vi "CT traits extraction_Maize stem_English version.vi"() -> ()   [LabVIEW 2015]
uses:
  <vilib>/Utility/file.llb/Write Delimited Spreadsheet (DBL).vi
  <vilib>/vision/NI_Vision_Development_Module.lvlib
  <vilib>/Utility/file.llb/Read From Spreadsheet File (string).vi
  CTThickness.dll
panel:
  out "Numeric":i32
  in  "Path of data storage":path=path "E:/文章投稿/51. 代明球老师-玉米胁迫实验/CT程序/section-test/results.txt"
  out "appended path":path
  in  "Path of reconstructed images":path=path "E:/文章投稿/51. 代明球老师-玉米胁迫实验/CT程序/section-test"
  out "Duty_cycle":dbl
  out "Cavity_area":dbl
  out "Hollow_area":dbl
  out "Vascular_area":dbl
  out "8. 维管束小区域图":T1(plugin-control)
  out "7. 维管束闭操作":T1(plugin-control)
  out "6. Vascular image":T1(plugin-control)
  out "5. Hollow grayscale image":T1(plugin-control)
  out "Culm_area":sgl
  out "Culm_wall_area":sgl
  out "Major_axis":sgl
  out "Minor_axis":sgl
  out "4. Hollow binary image":T1(plugin-control)
  out "Culm_diameter":sgl
  out "3. Culm wall image":T1(plugin-control)
  in  "图片路径 2":path=path "E:/文章投稿/51. 代明球老师-玉米胁迫实验/CT程序/CTThickness_2/空图.png"
  out "2. Culm wall image":T1(plugin-control)
  out "Wall_thickness":sgl
  out "1. Reconstructed transverse section images":T1(plugin-control)
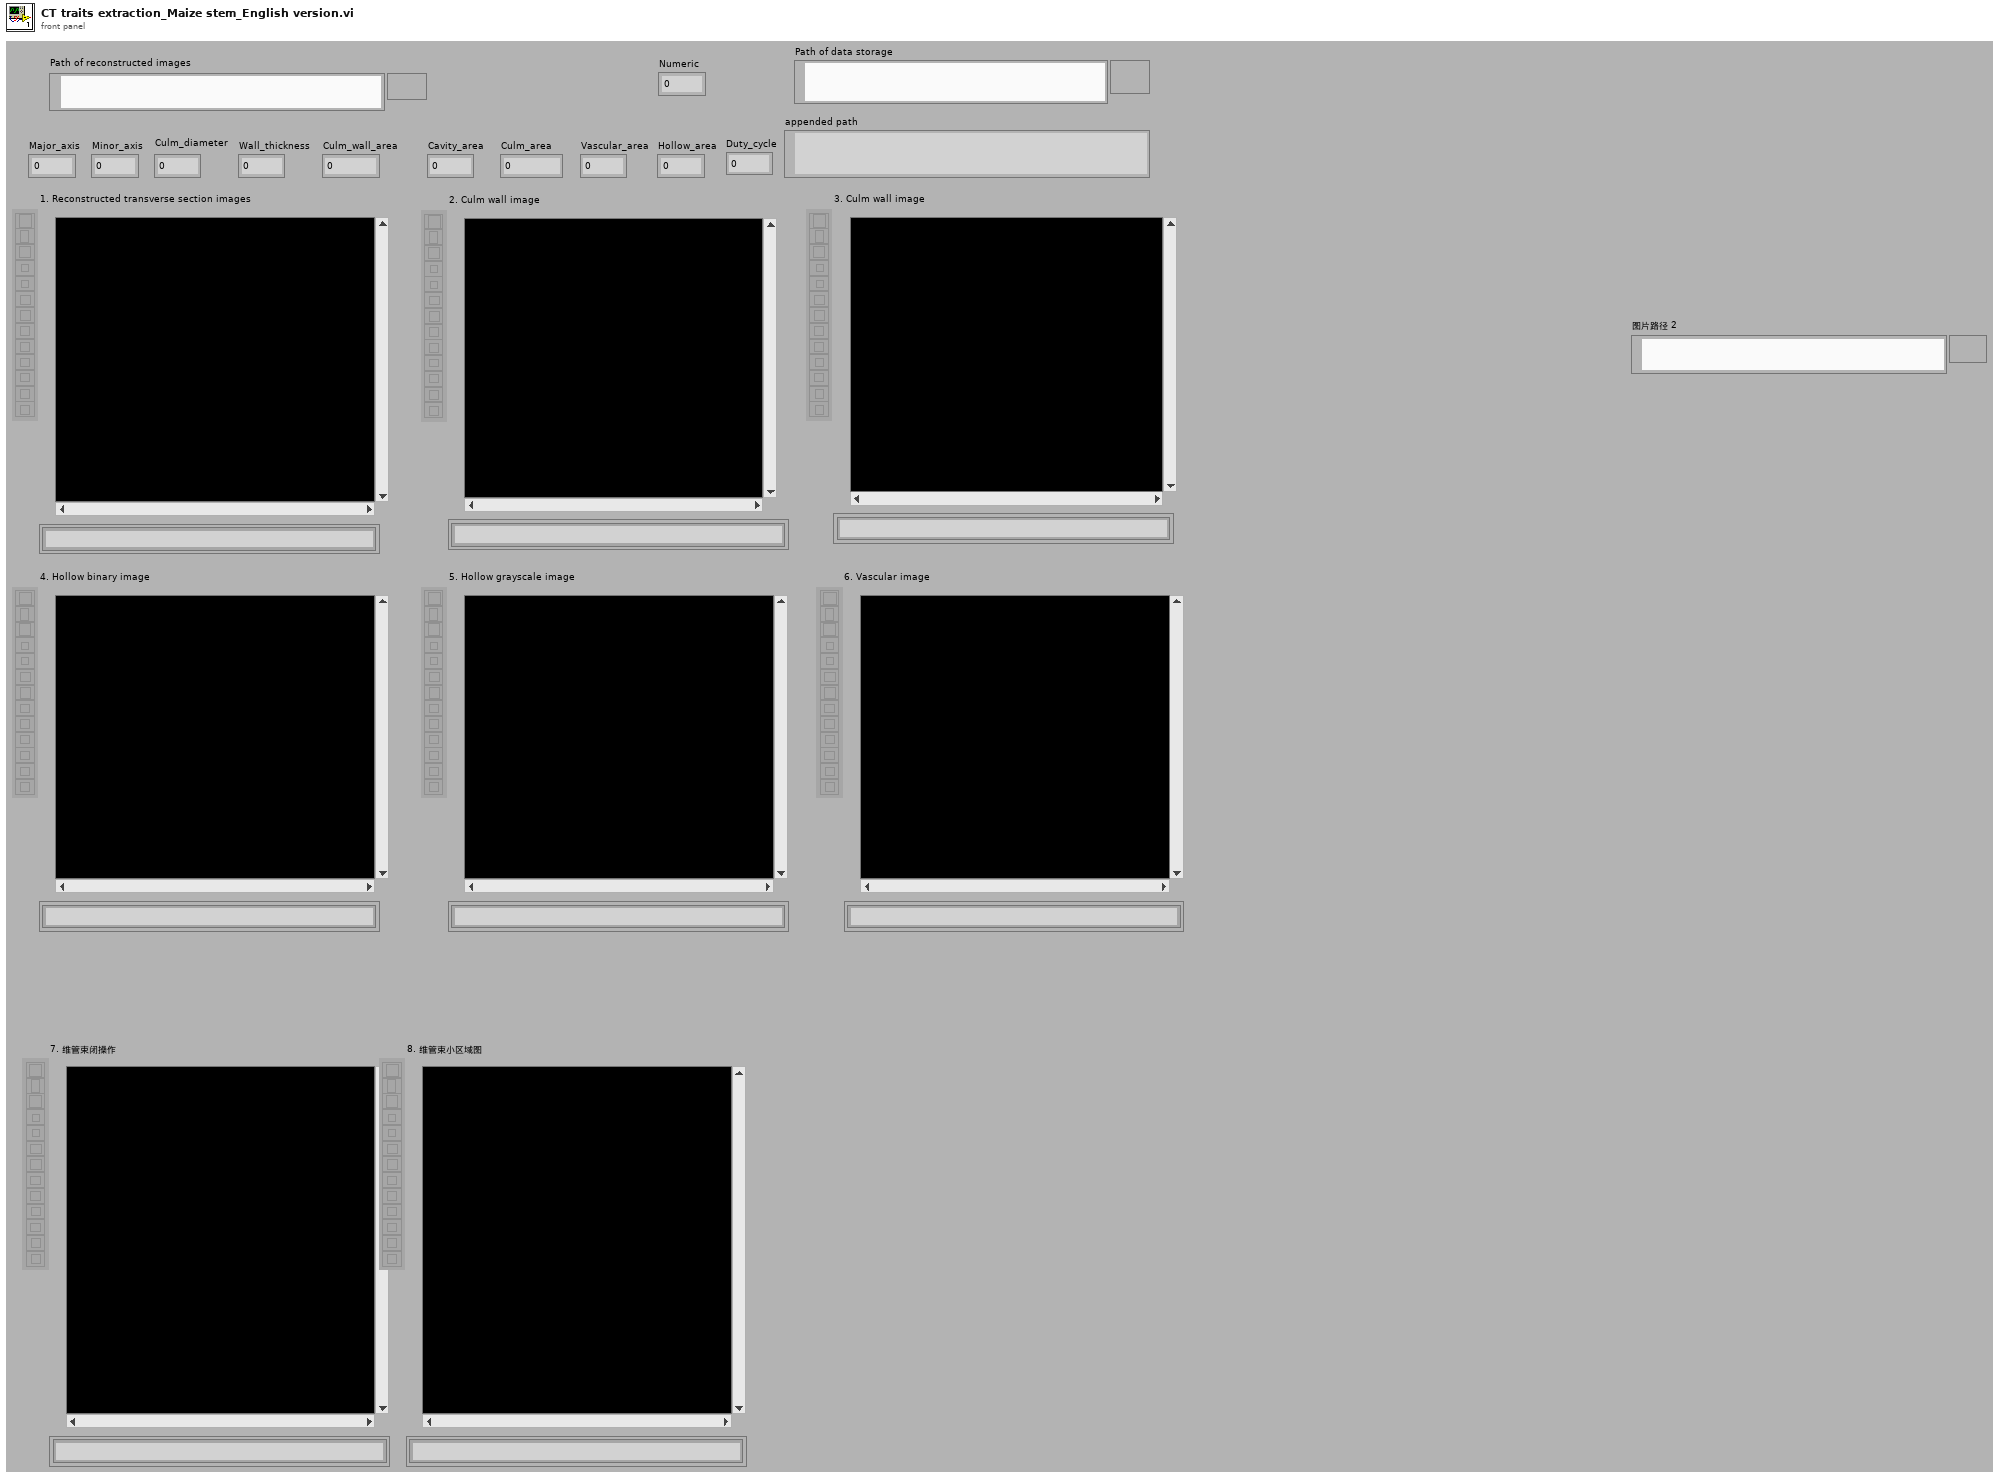
[diagram p1: front panel]
types:
  T1 = typedef "IMAQ Image.ctl" = refnum<image>
  T2 = enum32{"AutoM", "Close", "Dilate", "Erode", "Gradient", "Gradient in", "Gradient out", "HitMiss", "Open", "PClose", "POpen", "Thick", "Thin"}
  T3 = typedef "Particle Parameters" = i32
  T4 = typedef "Image Type" = u32
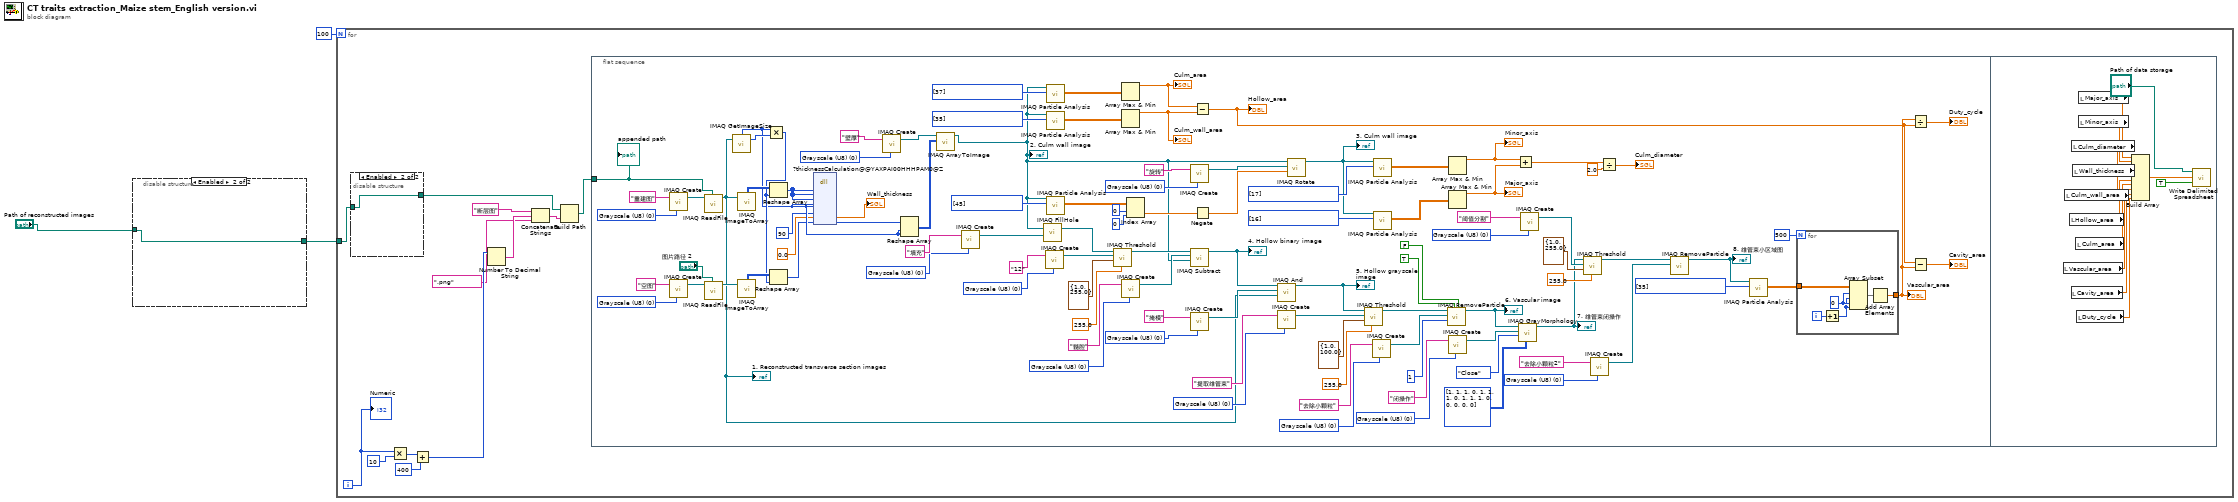
[diagram p0: block diagram]
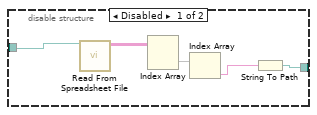
[diagram p2: hidden frame]
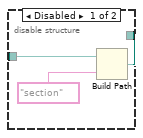
[diagram p3: hidden frame]
diagram:
  n1 = disable-structure shown="Enabled" {
    disable-tunnel: "Path of reconstructed images" -> [w8 w9]
    disable-tunnel: [w4 w9] -> w1
    frame Disabled {
      n2 = call-poly <vilib>:"Read From Spreadsheet File.vi"("file path (dialog if empty)"=w8) -> ("all rows"=w6:string[][])  [unwired: 3 in, 7 out]
      n3 = Index Array(array=w6) -> (element=w7:string[])  [unwired: 2 in]
      n4 = Index Array(array=w7) -> (element=w5:string)  [unwired: 1 in]
      n5 = String To Path(string=w5) -> (path=w4:path)
    }
    frame Enabled {
    }
  }
  n6 = for {
    N: 100 -> [_]
    tunnel: w1 -> [w12]
    i -> [w19]
    n7 = disable-structure shown="Enabled" {
      disable-tunnel: w12 -> [w24 w25]
      disable-tunnel: [w22 w25] -> w11
      frame Disabled {
        n8 = Build Path(base path=w24, name or relative path="section" ("string")) -> (appended path=w22:path)
      }
      frame Enabled {
      }
    }
    n9 = Multiply(x=w19, y=10) -> (x*y=w17:i32)
    n10 = Add(x=w17, y=400) -> (x+y=w15:i32)
    n11 = Number To Decimal String(number=w15) -> (decimal integer string=w21:string)  [unwired: 1 out]
    n12 = Concatenate Strings("断层图" ("string"), w21, ".png" ("string")) -> (w20:string)
    n13 = Build Path(base path=w11, name or relative path=w20) -> (appended path=w14:path)
    n14 = flat-sequence {
      tunnel: w14 -> [w37]
      frame #0 {
        w47 = T3[] [35] items=["Center of Mass X", "Center of Mass Y", "First Pixel X", "First Pixel Y", "Bounding Rect Left", "Bounding Rect Top", "Bounding Rect Right", "Bounding Rect Bottom", "Max Feret Diameter Start X", "Max Feret Diameter Start Y", "Max Feret Diameter End X", "Max Feret Diameter End Y", "Max Horiz. Segment Length Left", "Max Horiz. Segment Length Right", "Max Horiz. Segment Length Row", "-", "Bounding Rect Width", "Bounding Rect Height", "Bounding Rect Diagonal", "Perimeter", "Convex Hull Perimeter", "Holes' Perimeter", "Max Feret Diameter", "Equivalent Ellipse Major Axis", "Equivalent Ellipse Minor Axis", "Equivalent Ellipse Minor Axis (Feret)", "Equivalent Rect Long Side", "Equivalent Rect Short Side", "Equivalent Rect Diagonal", "Equivalent Rect Short Side (Feret)", "Average Horiz. Segment Length", "Average Vert. Segment Length", "Hydraulic Radius", "Waddel Disk Diameter", "-", "Area", "Holes' Area", "Particle & Holes' Area", "Convex Hull Area", "Image Area", "-", "Number of Holes", "Number of Horiz. Segments", "Number of Vert. Segments", "-", "Orientation", "Max Feret Diameter Orientation", "-", "% Area/Image Area", "% Area/(Particle & Holes' Area)", "Ratio of Equivalent Ellipse Axes", "Ratio of Equivalent Rect Sides", "-", "Elongation Factor", "Compactness Factor", "Heywood Circularity Factor", "Type Factor", "-", "Sum X", "Sum Y", "Sum XX", "Sum XY", "Sum YY", "Sum XXX", "Sum XXY", "Sum XYY", "Sum YYY", "-", "Moment of Inertia XX", "Moment of Inertia XY", "Moment of Inertia YY", "Moment of Inertia XXX", "Moment of Inertia XXY", "Moment of Inertia XYY", "Moment of Inertia YYY", "Norm. Moment of Inertia XX", "Norm. Moment of Inertia XY", "Norm. Moment of Inertia YY", "Norm. Moment of Inertia XXX", "Norm. Moment of Inertia XXY", "Norm. Moment of Inertia XYY", "Norm. Moment of Inertia YYY", "Hu Moment 1", "Hu Moment 2", "Hu Moment 3", "Hu Moment 4", "Hu Moment 5", "Hu Moment 6", "Hu Moment 7"] ("Pixel Measurements")
        w52 = T4 0 items=["Grayscale (U8)", "Grayscale (I16)", "Grayscale (SGL)", "Complex (CSG)", "RGB (U32)", "HSL (U32)", "RGB (U64)", "Grayscale (U16)"] ("Image Type")
        w58 = T4 0 items=["Grayscale (U8)", "Grayscale (I16)", "Grayscale (SGL)", "Complex (CSG)", "RGB (U32)", "HSL (U32)", "RGB (U64)", "Grayscale (U16)"] ("Image Type")
        w62 = T4 0 items=["Grayscale (U8)", "Grayscale (I16)", "Grayscale (SGL)", "Complex (CSG)", "RGB (U32)", "HSL (U32)", "RGB (U64)", "Grayscale (U16)"] ("Image Type")
        w73 = T4 0 items=["Grayscale (U8)", "Grayscale (I16)", "Grayscale (SGL)", "Complex (CSG)", "RGB (U32)", "HSL (U32)", "RGB (U64)", "Grayscale (U16)"] ("Image Type")
        w75 = T4 0 items=["Grayscale (U8)", "Grayscale (I16)", "Grayscale (SGL)", "Complex (CSG)", "RGB (U32)", "HSL (U32)", "RGB (U64)", "Grayscale (U16)"] ("Image Type")
        w78 = T4 0 items=["Grayscale (U8)", "Grayscale (I16)", "Grayscale (SGL)", "Complex (CSG)", "RGB (U32)", "HSL (U32)", "RGB (U64)", "Grayscale (U16)"] ("Image Type")
        w82 = T3[] [37] items=["Center of Mass X", "Center of Mass Y", "First Pixel X", "First Pixel Y", "Bounding Rect Left", "Bounding Rect Top", "Bounding Rect Right", "Bounding Rect Bottom", "Max Feret Diameter Start X", "Max Feret Diameter Start Y", "Max Feret Diameter End X", "Max Feret Diameter End Y", "Max Horiz. Segment Length Left", "Max Horiz. Segment Length Right", "Max Horiz. Segment Length Row", "-", "Bounding Rect Width", "Bounding Rect Height", "Bounding Rect Diagonal", "Perimeter", "Convex Hull Perimeter", "Holes' Perimeter", "Max Feret Diameter", "Equivalent Ellipse Major Axis", "Equivalent Ellipse Minor Axis", "Equivalent Ellipse Minor Axis (Feret)", "Equivalent Rect Long Side", "Equivalent Rect Short Side", "Equivalent Rect Diagonal", "Equivalent Rect Short Side (Feret)", "Average Horiz. Segment Length", "Average Vert. Segment Length", "Hydraulic Radius", "Waddel Disk Diameter", "-", "Area", "Holes' Area", "Particle & Holes' Area", "Convex Hull Area", "Image Area", "-", "Number of Holes", "Number of Horiz. Segments", "Number of Vert. Segments", "-", "Orientation", "Max Feret Diameter Orientation", "-", "% Area/Image Area", "% Area/(Particle & Holes' Area)", "Ratio of Equivalent Ellipse Axes", "Ratio of Equivalent Rect Sides", "-", "Elongation Factor", "Compactness Factor", "Heywood Circularity Factor", "Type Factor", "-", "Sum X", "Sum Y", "Sum XX", "Sum XY", "Sum YY", "Sum XXX", "Sum XXY", "Sum XYY", "Sum YYY", "-", "Moment of Inertia XX", "Moment of Inertia XY", "Moment of Inertia YY", "Moment of Inertia XXX", "Moment of Inertia XXY", "Moment of Inertia XYY", "Moment of Inertia YYY", "Norm. Moment of Inertia XX", "Norm. Moment of Inertia XY", "Norm. Moment of Inertia YY", "Norm. Moment of Inertia XXX", "Norm. Moment of Inertia XXY", "Norm. Moment of Inertia XYY", "Norm. Moment of Inertia YYY", "Hu Moment 1", "Hu Moment 2", "Hu Moment 3", "Hu Moment 4", "Hu Moment 5", "Hu Moment 6", "Hu Moment 7"] ("Pixel Measurements")
        w84 = T3[] [35] items=["Center of Mass X", "Center of Mass Y", "First Pixel X", "First Pixel Y", "Bounding Rect Left", "Bounding Rect Top", "Bounding Rect Right", "Bounding Rect Bottom", "Max Feret Diameter Start X", "Max Feret Diameter Start Y", "Max Feret Diameter End X", "Max Feret Diameter End Y", "Max Horiz. Segment Length Left", "Max Horiz. Segment Length Right", "Max Horiz. Segment Length Row", "-", "Bounding Rect Width", "Bounding Rect Height", "Bounding Rect Diagonal", "Perimeter", "Convex Hull Perimeter", "Holes' Perimeter", "Max Feret Diameter", "Equivalent Ellipse Major Axis", "Equivalent Ellipse Minor Axis", "Equivalent Ellipse Minor Axis (Feret)", "Equivalent Rect Long Side", "Equivalent Rect Short Side", "Equivalent Rect Diagonal", "Equivalent Rect Short Side (Feret)", "Average Horiz. Segment Length", "Average Vert. Segment Length", "Hydraulic Radius", "Waddel Disk Diameter", "-", "Area", "Holes' Area", "Particle & Holes' Area", "Convex Hull Area", "Image Area", "-", "Number of Holes", "Number of Horiz. Segments", "Number of Vert. Segments", "-", "Orientation", "Max Feret Diameter Orientation", "-", "% Area/Image Area", "% Area/(Particle & Holes' Area)", "Ratio of Equivalent Ellipse Axes", "Ratio of Equivalent Rect Sides", "-", "Elongation Factor", "Compactness Factor", "Heywood Circularity Factor", "Type Factor", "-", "Sum X", "Sum Y", "Sum XX", "Sum XY", "Sum YY", "Sum XXX", "Sum XXY", "Sum XYY", "Sum YYY", "-", "Moment of Inertia XX", "Moment of Inertia XY", "Moment of Inertia YY", "Moment of Inertia XXX", "Moment of Inertia XXY", "Moment of Inertia XYY", "Moment of Inertia YYY", "Norm. Moment of Inertia XX", "Norm. Moment of Inertia XY", "Norm. Moment of Inertia YY", "Norm. Moment of Inertia XXX", "Norm. Moment of Inertia XXY", "Norm. Moment of Inertia XYY", "Norm. Moment of Inertia YYY", "Hu Moment 1", "Hu Moment 2", "Hu Moment 3", "Hu Moment 4", "Hu Moment 5", "Hu Moment 6", "Hu Moment 7"] ("Pixel Measurements")
        w93 = T4 0 items=["Grayscale (U8)", "Grayscale (I16)", "Grayscale (SGL)", "Complex (CSG)", "RGB (U32)", "HSL (U32)", "RGB (U64)", "Grayscale (U16)"] ("Image Type")
        w96 = T4 0 items=["Grayscale (U8)", "Grayscale (I16)", "Grayscale (SGL)", "Complex (CSG)", "RGB (U32)", "HSL (U32)", "RGB (U64)", "Grayscale (U16)"] ("Image Type")
        w98 = T4 0 items=["Grayscale (U8)", "Grayscale (I16)", "Grayscale (SGL)", "Complex (CSG)", "RGB (U32)", "HSL (U32)", "RGB (U64)", "Grayscale (U16)"] ("Image Type")
        w107 = T3[] [45] items=["Center of Mass X", "Center of Mass Y", "First Pixel X", "First Pixel Y", "Bounding Rect Left", "Bounding Rect Top", "Bounding Rect Right", "Bounding Rect Bottom", "Max Feret Diameter Start X", "Max Feret Diameter Start Y", "Max Feret Diameter End X", "Max Feret Diameter End Y", "Max Horiz. Segment Length Left", "Max Horiz. Segment Length Right", "Max Horiz. Segment Length Row", "-", "Bounding Rect Width", "Bounding Rect Height", "Bounding Rect Diagonal", "Perimeter", "Convex Hull Perimeter", "Holes' Perimeter", "Max Feret Diameter", "Equivalent Ellipse Major Axis", "Equivalent Ellipse Minor Axis", "Equivalent Ellipse Minor Axis (Feret)", "Equivalent Rect Long Side", "Equivalent Rect Short Side", "Equivalent Rect Diagonal", "Equivalent Rect Short Side (Feret)", "Average Horiz. Segment Length", "Average Vert. Segment Length", "Hydraulic Radius", "Waddel Disk Diameter", "-", "Area", "Holes' Area", "Particle & Holes' Area", "Convex Hull Area", "Image Area", "-", "Number of Holes", "Number of Horiz. Segments", "Number of Vert. Segments", "-", "Orientation", "Max Feret Diameter Orientation", "-", "% Area/Image Area", "% Area/(Particle & Holes' Area)", "Ratio of Equivalent Ellipse Axes", "Ratio of Equivalent Rect Sides", "-", "Elongation Factor", "Compactness Factor", "Heywood Circularity Factor", "Type Factor", "-", "Sum X", "Sum Y", "Sum XX", "Sum XY", "Sum YY", "Sum XXX", "Sum XXY", "Sum XYY", "Sum YYY", "-", "Moment of Inertia XX", "Moment of Inertia XY", "Moment of Inertia YY", "Moment of Inertia XXX", "Moment of Inertia XXY", "Moment of Inertia XYY", "Moment of Inertia YYY", "Norm. Moment of Inertia XX", "Norm. Moment of Inertia XY", "Norm. Moment of Inertia YY", "Norm. Moment of Inertia XXX", "Norm. Moment of Inertia XXY", "Norm. Moment of Inertia XYY", "Norm. Moment of Inertia YYY", "Hu Moment 1", "Hu Moment 2", "Hu Moment 3", "Hu Moment 4", "Hu Moment 5", "Hu Moment 6", "Hu Moment 7"] ("Pixel Measurements")
        w109 = T4 0 items=["Grayscale (U8)", "Grayscale (I16)", "Grayscale (SGL)", "Complex (CSG)", "RGB (U32)", "HSL (U32)", "RGB (U64)", "Grayscale (U16)"] ("Image Type")
        w115 = T3[] [17] items=["Center of Mass X", "Center of Mass Y", "First Pixel X", "First Pixel Y", "Bounding Rect Left", "Bounding Rect Top", "Bounding Rect Right", "Bounding Rect Bottom", "Max Feret Diameter Start X", "Max Feret Diameter Start Y", "Max Feret Diameter End X", "Max Feret Diameter End Y", "Max Horiz. Segment Length Left", "Max Horiz. Segment Length Right", "Max Horiz. Segment Length Row", "-", "Bounding Rect Width", "Bounding Rect Height", "Bounding Rect Diagonal", "Perimeter", "Convex Hull Perimeter", "Holes' Perimeter", "Max Feret Diameter", "Equivalent Ellipse Major Axis", "Equivalent Ellipse Minor Axis", "Equivalent Ellipse Minor Axis (Feret)", "Equivalent Rect Long Side", "Equivalent Rect Short Side", "Equivalent Rect Diagonal", "Equivalent Rect Short Side (Feret)", "Average Horiz. Segment Length", "Average Vert. Segment Length", "Hydraulic Radius", "Waddel Disk Diameter", "-", "Area", "Holes' Area", "Particle & Holes' Area", "Convex Hull Area", "Image Area", "-", "Number of Holes", "Number of Horiz. Segments", "Number of Vert. Segments", "-", "Orientation", "Max Feret Diameter Orientation", "-", "% Area/Image Area", "% Area/(Particle & Holes' Area)", "Ratio of Equivalent Ellipse Axes", "Ratio of Equivalent Rect Sides", "-", "Elongation Factor", "Compactness Factor", "Heywood Circularity Factor", "Type Factor", "-", "Sum X", "Sum Y", "Sum XX", "Sum XY", "Sum YY", "Sum XXX", "Sum XXY", "Sum XYY", "Sum YYY", "-", "Moment of Inertia XX", "Moment of Inertia XY", "Moment of Inertia YY", "Moment of Inertia XXX", "Moment of Inertia XXY", "Moment of Inertia XYY", "Moment of Inertia YYY", "Norm. Moment of Inertia XX", "Norm. Moment of Inertia XY", "Norm. Moment of Inertia YY", "Norm. Moment of Inertia XXX", "Norm. Moment of Inertia XXY", "Norm. Moment of Inertia XYY", "Norm. Moment of Inertia YYY", "Hu Moment 1", "Hu Moment 2", "Hu Moment 3", "Hu Moment 4", "Hu Moment 5", "Hu Moment 6", "Hu Moment 7"] ("Pixel Measurements")
        w116 = T3[] [16] items=["Center of Mass X", "Center of Mass Y", "First Pixel X", "First Pixel Y", "Bounding Rect Left", "Bounding Rect Top", "Bounding Rect Right", "Bounding Rect Bottom", "Max Feret Diameter Start X", "Max Feret Diameter Start Y", "Max Feret Diameter End X", "Max Feret Diameter End Y", "Max Horiz. Segment Length Left", "Max Horiz. Segment Length Right", "Max Horiz. Segment Length Row", "-", "Bounding Rect Width", "Bounding Rect Height", "Bounding Rect Diagonal", "Perimeter", "Convex Hull Perimeter", "Holes' Perimeter", "Max Feret Diameter", "Equivalent Ellipse Major Axis", "Equivalent Ellipse Minor Axis", "Equivalent Ellipse Minor Axis (Feret)", "Equivalent Rect Long Side", "Equivalent Rect Short Side", "Equivalent Rect Diagonal", "Equivalent Rect Short Side (Feret)", "Average Horiz. Segment Length", "Average Vert. Segment Length", "Hydraulic Radius", "Waddel Disk Diameter", "-", "Area", "Holes' Area", "Particle & Holes' Area", "Convex Hull Area", "Image Area", "-", "Number of Holes", "Number of Horiz. Segments", "Number of Vert. Segments", "-", "Orientation", "Max Feret Diameter Orientation", "-", "% Area/Image Area", "% Area/(Particle & Holes' Area)", "Ratio of Equivalent Ellipse Axes", "Ratio of Equivalent Rect Sides", "-", "Elongation Factor", "Compactness Factor", "Heywood Circularity Factor", "Type Factor", "-", "Sum X", "Sum Y", "Sum XX", "Sum XY", "Sum YY", "Sum XXX", "Sum XXY", "Sum XYY", "Sum YYY", "-", "Moment of Inertia XX", "Moment of Inertia XY", "Moment of Inertia YY", "Moment of Inertia XXX", "Moment of Inertia XXY", "Moment of Inertia XYY", "Moment of Inertia YYY", "Norm. Moment of Inertia XX", "Norm. Moment of Inertia XY", "Norm. Moment of Inertia YY", "Norm. Moment of Inertia XXX", "Norm. Moment of Inertia XXY", "Norm. Moment of Inertia XYY", "Norm. Moment of Inertia YYY", "Hu Moment 1", "Hu Moment 2", "Hu Moment 3", "Hu Moment 4", "Hu Moment 5", "Hu Moment 6", "Hu Moment 7"] ("Pixel Measurements")
        w120 = T4 0 items=["Grayscale (U8)", "Grayscale (I16)", "Grayscale (SGL)", "Complex (CSG)", "RGB (U32)", "HSL (U32)", "RGB (U64)", "Grayscale (U16)"] ("Image Type")
        w125 = T4 0 items=["Grayscale (U8)", "Grayscale (I16)", "Grayscale (SGL)", "Complex (CSG)", "RGB (U32)", "HSL (U32)", "RGB (U64)", "Grayscale (U16)"] ("Image Type")
        w128 = T4 0 items=["Grayscale (U8)", "Grayscale (I16)", "Grayscale (SGL)", "Complex (CSG)", "RGB (U32)", "HSL (U32)", "RGB (U64)", "Grayscale (U16)"] ("Image Type")
        n15 = call "IMAQ Create"("Image Name"="重建图", "Image Type"=w128) -> ("New Image"=w129:T1)  [unwired: 2 in, 2 out]
        n16 = call "IMAQ Create"("Image Name"="空图", "Image Type"=w120) -> ("New Image"=w122:T1)  [unwired: 2 in, 2 out]
        n17 = call "IMAQ ReadFile"("File Path"=w37, "Image"=w129) -> ("Image Out"=w36:T1)  [unwired: 3 in, 6 out]
        "1. Reconstructed transverse section images" <- w36
        n18 = call "IMAQ ReadFile"("File Path"="图片路径 2", "Image"=w122) -> ("Image Out"=w119:T1)  [unwired: 3 in, 6 out]
        n19 = call "IMAQ GetImageSize"("Image"=w36) -> ("Y Resolution"=w35:i32, "X Resolution"=w32:i32)  [unwired: 1 in, 3 out]
        n20 = call "IMAQ ImageToArray"("Image"=w36) -> ("Image Pixels (U8)"=w127:u8[][])  [unwired: 2 in, 5 out]
        n21 = call "IMAQ ImageToArray"("Image"=w119) -> ("Image Pixels (U8)"=w118:u8[][])  [unwired: 2 in, 5 out]
        n22 = Multiply(x=w32, y=w35) -> (x*y=w34:i32)
        n23 = Reshape Array(w127, w34) -> (w33:u8[])
        n24 = Reshape Array(w118, w34) -> (w29:u8[])
        n25 = dll-call lib="PTH2gabs E文章投稿&51. 代明球老师-玉米胁迫实验CT程序\nCTThickness_2CTThickness.dll" fn="?thicknessCalculation@@YAXPAI00HHHPAM0@Z"("R"=w33, "G"=w33, "B"=w33, "ROW"=w32, "COL"=w32, "INPUT GRAY"=90 ("grayScale"), "AVERAGE THICKNESS"=sgl 0.0 ("averageThickness"), "IMAGE"=w29) -> ("AVERAGE THICKNESS"=→"Wall_thickness":sgl, "IMAGE"=w27:i8[])  [unwired: 7 in, 5 out]
        n26 = call "IMAQ Create"("Image Name"="壁厚", "Image Type"=w125) -> ("New Image"=w124:T1)  [unwired: 2 in, 2 out]
        n27 = Reshape Array(w27, w32, w32) -> (w117:i8[][])
        n28 = call "IMAQ ArrayToImage"("Image Pixels (U8)"=w117, "Image"=w124) -> ("Image Out"=w26:T1)  [unwired: 4 in, 5 out]
        "2. Culm wall image" <- w26
        n29 = call "IMAQ Create"("Image Name"="填充", "Image Type"=w96) -> ("New Image"=w95:T1)  [unwired: 2 in, 2 out]
        n30 = call "IMAQ FillHole"("Image Dst"=w95, "Image Src"=w26) -> ("Image Dst Out"=w89:T1)  [unwired: 2 in, 3 out]
        n31 = call "IMAQ Create"("Image Name"="12", "Image Type"=w93) -> ("New Image"=w92:T1)  [unwired: 2 in, 2 out]
        n32 = call "IMAQ Particle Analysis"("Pixel Measurements"=w82, "Image"=w26) -> ("Particle Measurements (Pixels)"=w81:dbl[][])  [unwired: 3 in, 6 out]
        n33 = call "IMAQ Particle Analysis"("Pixel Measurements"=w84, "Image"=w26) -> ("Particle Measurements (Pixels)"=w83:dbl[][])  [unwired: 3 in, 6 out]
        n34 = call "IMAQ Particle Analysis"("Pixel Measurements"=w107, "Image"=w26) -> ("Particle Measurements (Pixels)"=w103:dbl[][])  [unwired: 3 in, 6 out]
        n35 = call "IMAQ Threshold"("Replace Value"=sgl 255.0, "Range"=cluster{"Lower value":sgl, "Upper value":sgl} {"Lower value"=1.0, "Upper value"=255.0}, "Image Dst"=w92, "Image Src"=w89) -> ("Image Dst Out"=w88:T1)  [unwired: 2 in, 5 out]
        n36 = Array Max & Min(array=w81) -> (max value=w44:dbl)  [unwired: 3 out]
        "Culm_area" <- w44
        n37 = Array Max & Min(array=w83) -> (max value=w43:dbl)  [unwired: 3 out]
        "Culm_wall_area" <- w43
        n38 = call "IMAQ Create"("Image Name"="髓腔", "Image Type"=w98) -> ("New Image"=w87:T1)  [unwired: 2 in, 2 out]
        n39 = Index Array(array=w103, index (row)=0, index (col)=0 ("disabled index (col)")) -> (element=w104:dbl)
        n40 = call "IMAQ Create"("Image Name"="旋转", "Image Type"=w109) -> ("New Image"=w108:T1)  [unwired: 2 in, 2 out]
        n41 = call "IMAQ Subtract"("Image Src A"=w88, "Image Dst"=w87, "Image Src B"=w26) -> ("Image Dst Out"=w80:T1)  [unwired: 2 in, 3 out]
        "4. Hollow binary image" <- w80
        n42 = call "IMAQ Create"("Image Name"="掩模", "Image Type"=w78) -> ("New Image"=w77:T1)  [unwired: 2 in, 2 out]
        n43 = Subtract(x=w44, y=w43) -> (x-y=w40:dbl)
        "Hollow_area" <- w40
        n44 = Negate(x=w104) -> (-x=w102:dbl)
        n45 = call "IMAQ And"("Image Src B"=w36, "Image Dst"=w77, "Image Src A"=w80) -> ("Image Dst Out"=w67:T1)  [unwired: 3 in, 5 out]
        "5. Hollow grayscale image" <- w67
        n46 = call "IMAQ Create"("Image Name"="提取维管束", "Image Type"=w75) -> ("New Image"=w68:T1)  [unwired: 2 in, 2 out]
        n47 = call "IMAQ Rotate"("Angle (degrees)"=w102, "Image Dst"=w108, "Image Src"=w26) -> ("Image Dst Out"=w101:T1)  [unwired: 5 in, 3 out]
        "3. Culm wall image" <- w101
        n48 = call "IMAQ Threshold"("Replace Value"=sgl 255.0, "Range"=cluster{"Lower value":sgl, "Upper value":sgl} {"Lower value"=1.0, "Upper value"=100.0}, "Image Dst"=w68, "Image Src"=w67) -> ("Image Dst Out"=w65:T1)  [unwired: 2 in, 5 out]
        n49 = call "IMAQ Create"("Image Name"="去除小颗粒", "Image Type"=w73) -> ("New Image"=w72:T1)  [unwired: 2 in, 2 out]
        n50 = call "IMAQ Particle Analysis"("Pixel Measurements"=w115, "Image"=w101) -> ("Particle Measurements (Pixels)"=w114:dbl[][])  [unwired: 3 in, 6 out]
        n51 = call "IMAQ Particle Analysis"("Pixel Measurements"=w116, "Image"=w101) -> ("Particle Measurements (Pixels)"=w113:dbl[][])  [unwired: 3 in, 6 out]
        n52 = call "IMAQ RemoveParticle"("Connectivity 4/8 (8)"=FALSE, "Square/Hexa (Square)"=TRUE, "Number of Erosion"=1, "Image Dst"=w72, "Image Src"=w65) -> ("Image Dst Out"=w64:T1)  [unwired: 2 in, 4 out]
        "6. Vascular image" <- w64
        n53 = Array Max & Min(array=w114) -> (max value=w86:dbl)  [unwired: 3 out]
        "Minor_axis" <- w86
        n54 = Array Max & Min(array=w113) -> (max value=w85:dbl)  [unwired: 3 out]
        "Major_axis" <- w85
        n55 = call "IMAQ Create"("Image Name"="闭操作", "Image Type"=w62) -> ("New Image"=w61:T1)  [unwired: 2 in, 2 out]
        n56 = Add(x=w86, y=w85) -> (x+y=w112:dbl)
        n57 = call "IMAQ GrayMorphology"("Structuring Element"=i32[][] [[1, 1, 1, 0], [1, 1, 1, 0], [1, 1, 1, 0], [0, 0, 0, 0]], "Operation"=T2."Close", "Image Dst"=w61, "Image Src"=w64) -> ("Image Dst Out"=w38:T1)  [unwired: 3 in, 4 out]
        "7. 维管束闭操作" <- w38
        n58 = call "IMAQ Create"("Image Name"="阈值分割", "Image Type"=w58) -> ("New Image"=w56:T1)  [unwired: 2 in, 2 out]
        n59 = call "IMAQ Threshold"("Replace Value"=sgl 255.0, "Range"=cluster{"Lower value":sgl, "Upper value":sgl} {"Lower value"=1.0, "Upper value"=255.0}, "Image Dst"=w56, "Image Src"=w38) -> ("Image Dst Out"=w53:T1)  [unwired: 2 in, 5 out]
        n60 = call "IMAQ Create"("Image Name"="去除小颗粒2", "Image Type"=w52) -> ("New Image"=w50:T1)  [unwired: 2 in, 2 out]
        n61 = Divide(x=w112, y=2.0) -> (x/y=→"Culm_diameter":dbl)
        n62 = call "IMAQ RemoveParticle"("Image Dst"=w50, "Image Src"=w53) -> ("Image Dst Out"=w48:T1)  [unwired: 5 in, 4 out]
        "8. 维管束小区域图" <- w48
        n63 = call "IMAQ Particle Analysis"("Pixel Measurements"=w47, "Image"=w48) -> ("Particle Measurements (Pixels)"=w46:dbl[][])  [unwired: 3 in, 6 out]
        n64 = for {
          N: 500 -> [_]
          tunnel: w46 -> [w135]
          tunnel: [w133] -> w41
          i -> [w136]
          w132 = 0 ("index")
          n65 = Increment(x=w136) -> (x+1=w131:i32)
          n66 = Array Subset(array=w135, index (row)=w132, length (row)=w131, index (col)=w132, length (col)=w131) -> (w134:dbl[][])
          n67 = Add Array Elements(numeric array=w134) -> (sum=w133:dbl)
        }
        "Vascular_area" <- w41
        n68 = Divide(x=w41, y=w40) -> (x/y=→"Duty_cycle":dbl)
        n69 = Subtract(x=w40, y=w41) -> (x-y=→"Cavity_area":dbl)
        "appended path" <- w37
      }
      frame #1 {
        n70 = local read "Vascular_area"() -> (w142:dbl)
        n71 = local read "Culm_wall_area"() -> (w145:sgl)
        n72 = local read "Hollow_area"() -> (w144:dbl)
        n73 = local read "Cavity_area"() -> (w141:dbl)
        n74 = local read "Culm_diameter"() -> (w147:sgl)
        n75 = local read "Wall_thickness"() -> (w146:sgl)
        n76 = local read "Culm_area"() -> (w143:sgl)
        n77 = local read "Duty_cycle"() -> (w140:dbl)
        n78 = local read "Major_axis"() -> (w149:sgl)
        n79 = local read "Minor_axis"() -> (w148:sgl)
        n80 = Build Array(w149, w148, w147, w146, w145, w144, w143, w142, w141, w140) -> (w138:dbl[])
        n81 = call-poly <vilib>:"Write Delimited Spreadsheet.vi"("file path (dialog if empty)"="Path of data storage", "1D data"=w138, "append to file? (F)"=TRUE ("append to file? (new file:F)")) -> ()  [unwired: 11 in, 2 out]
      }
    }
    "Numeric" <- w19
  }
